vi "ConnectionWriteData.vi"(8 "error in (no error)":errorcluster, 10 "DataToSend":refnum<class "DataToSend.lvclass">, 11 "Tcp in":refnum<class "Tcp.lvclass">) -> (0 "error out":errorcluster, 3 "Tcp out":refnum<class "Tcp.lvclass">)   [LabVIEW 2022 SP3, in "Tcp.lvlib" / "Tcp.lvclass"]
uses:
  Tcp.lvclass
  Tcp.lvclass/Tcp.ctl
  Connection/Connection Messages/WriteData Msg/WriteData Msg.lvclass
  DataToSend/DataToSend.lvclass
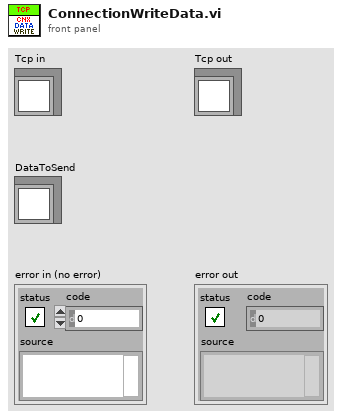
[diagram p1: front panel]
types:
  T1 = map{u64, refnum<class "Message Enqueuer.lvclass">}
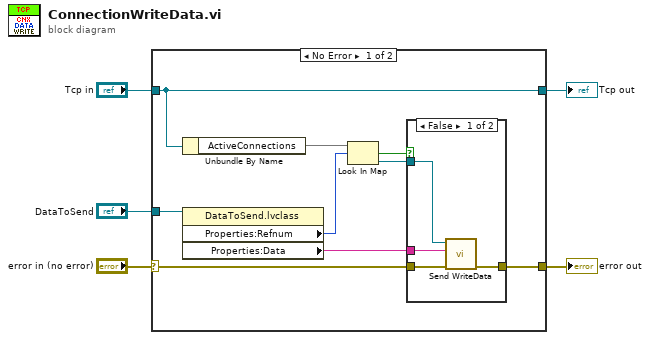
[diagram p0: block diagram]
diagram:
  n1 = case shown="No Error" "error in (no error)" {
    selector: "error in (no error)" -> [w14 w21]
    tunnel: [w9 w21] -> w4
    tunnel: [w13 w20] -> w2
    tunnel: "Tcp in" -> [w13 w20]
    tunnel: "DataToSend" -> [w11 _]
    frame No Error {
      n2 = Unbundle By Name(w13) -> ("ActiveConnections"=w12:T1)
      n3 = property class="DataToSend.lvclass"(reference=w11) -> ("Properties:Refnum"=w10:u64, "Properties:Data"=w7:string)  [unwired: 1 in, 2 out]
      n4 = Look In Map(map=w12, key=w10) -> (key not found?=w6:bool, value=w8:refnum<class "Message Enqueuer.lvclass">)  [unwired: 1 in]
      n5 = case shown="False" w6 {
        tunnel: w14 -> [w18 w19]
        tunnel: [w17 w19] -> w9
        tunnel: w8 -> [w16 _]
        tunnel: w7 -> [w15 _]
        frame False {
          n6 = call "Send WriteData.vi"("error in (no error)"=w18, "Data"=w15, "Message Enqueuer"=w16) -> ("error out"=w17:errorcluster)  [unwired: 7 in, 1 out]
        }
        frame True {
        }
      }
    }
    frame Error {
    }
  }
  "error out" <- w4
  "Tcp out" <- w2
